vi "ReadBytes.vi"(6 "Timeout (1000 ms)":u16=1000, 8 "error in (no error)":errorcluster, 9 "Bytes To Read":u8, 10 "Register Address":u8 format="%.0x", 11 "mainI2CDevice in":refnum<class "mainI2CDevice.lvclass">) -> (0 "error out":errorcluster, 2 "Data":u8[](array[numeric]), 3 "mainI2CDevice out":refnum<class "mainI2CDevice.lvclass">)   [LabVIEW 2020, in "RPI.lvlib" / "mainI2CDevice.lvclass"]
doc: "Read the specified number of bytes from the I2C slave."
uses:
  mainI2CDevice.lvclass
  mainI2CDevice.lvclass/mainI2CDevice.ctl
  <vilib>/MakerHub/LINX/Private/Local IO/LinxI2cWrite.vi
  <vilib>/MakerHub/LINX/Public/Utilities/Check Channel.vi
  <vilib>/MakerHub/LINX/Private/Local IO/Handle Errors.vi
  <vilib>/MakerHub/LINX/Private/Utilties/Generate Error.vi
  <vilib>/MakerHub/LINX/LMH-LINX.lvlib
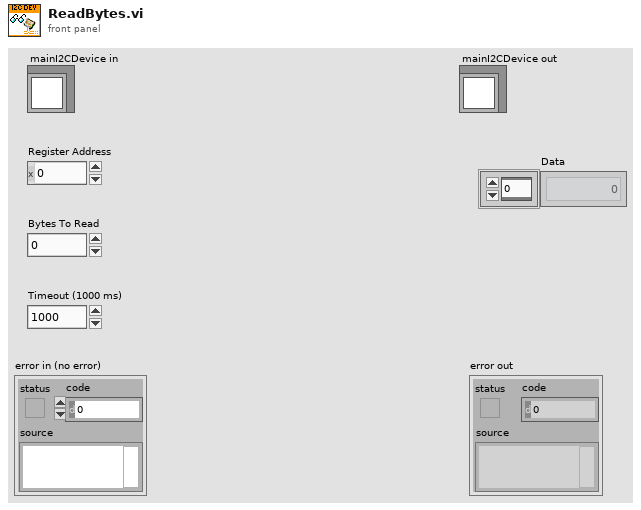
[diagram p1: front panel]
types:
  T1 = typedef "LMH-LINX.lvlib/LINX Ref.ctl" = cluster{"IO":T2, "Interface":T3, "LINX Device Config":T4}
  T2 = typedef "LMH-LINX.lvlib/Platform.ctl" = enum16{"Remote", "Local"}
  T3 = typedef "LMH-LINX.lvlib/Interface.ctl" = enum16{"Serial", "TCP"}
  T4 = typedef "LMH-LINX.lvlib/Device.lvlib/LINX Device Config.ctl" = cluster{"Interface":T3, "COM Port":refnum<visa-resource-name>, "TCP Configuration":T5, "Device Family":u8, "Device ID":u8, "Device Name":string, "TCP Ref":refnum<k5>, "Channels":T6}
  T5 = typedef "LMH-LINX.lvlib/Device.lvlib/TCP Config.ctl" = cluster{"IP Address":string, "Port":u16}
  T6 = typedef "LMH-LINX.lvlib/Channels.ctl" = cluster{"DI":u8[], "DO":u8[], "AI":u8[], "AO":u8[], "PWM":u8[], "QE":u8[], "UART":u8[], "I2C 2":u8[], "SPI":u8[], "CAN":u8[], "Servo":u8[], "AI Ref (V)":dbl, "AI Resolution (Bits)":u8, "AO Ref (V)":dbl, "AO Resolution (Bits)":u8}
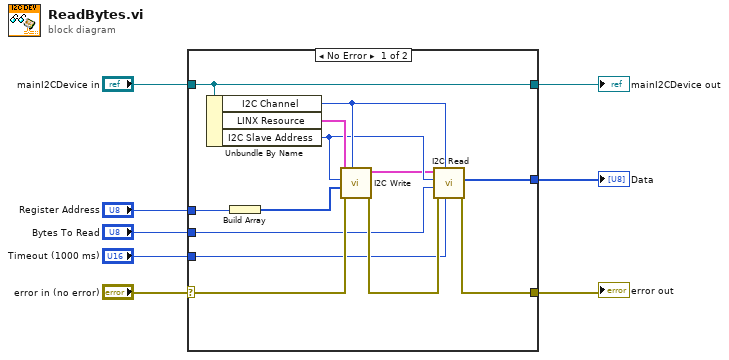
[diagram p0: block diagram]
diagram:
  n1 = case shown="No Error" "error in (no error)" {
    selector: "error in (no error)" -> [w15 w23]
    tunnel: [w20 w23] -> w7
    tunnel: [w21 w22] -> w5
    tunnel: "mainI2CDevice in" -> [w21 w22]
    tunnel: "Bytes To Read" -> [w11 _]
    tunnel: [w19 _] -> w3
    tunnel: "Register Address" -> [w13 _]
    tunnel: "Timeout (1000 ms)" -> [w9 _]
    frame No Error {
      n2 = Unbundle By Name(w21) -> ("I2C Channel"=w17:u8, "LINX Resource"=w18:T1, "I2C Slave Address"=w16:u8)
      n3 = Build Array(w13) -> (w12:u8[])
      n4 = call <vilib>:"I2C Write.vi"("I2C Channel"=w17, "Error In"=w15, "Data"=w12, "I2C Slave Address (0)"=w16, "LINX Resource"=w18) -> ("Error Out"=w14:errorcluster, "LINX Resource"=w10:T1)  [unwired: 5 in]
      n5 = call <vilib>:"I2C Read.vi"("Timeout (1000 ms)"=w9, "I2C Channel"=w17, "Error In"=w14, "Bytes To Read"=w11, "I2C Slave Address (0)"=w16, "LINX Resource"=w10) -> ("Error Out"=w20:errorcluster, "Data"=w19:u8[])  [unwired: 3 in, 1 out]
    }
    frame Error {
    }
  }
  "error out" <- w7
  "mainI2CDevice out" <- w5
  "Data" <- w3
